vi "FindAllMessages.vi"(8 "error in (no error)":errorcluster, 11 "CS++Actor in":refnum<class "CS++Actor.lvclass">) -> (0 "error out":errorcluster, 3 "CS++Actor out":refnum<class "CS++Actor.lvclass">)   [LabVIEW 2014, in "CS++Actor.lvlib" / "CS++Actor.lvclass"]
doc: "Searches for all messages in this actor."
uses:
  CS++Actor.lvclass
  CS++Actor.lvclass/CS++Actor.ctl
  CSPP_Message/CS++Message.lvclass
  CSPP_Message/CS++Message.lvclass/CS++Message.ctl
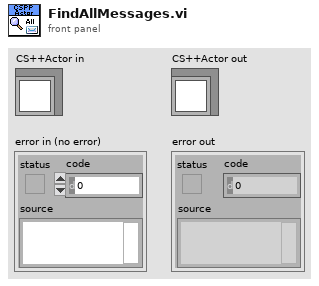
[diagram p1: front panel]
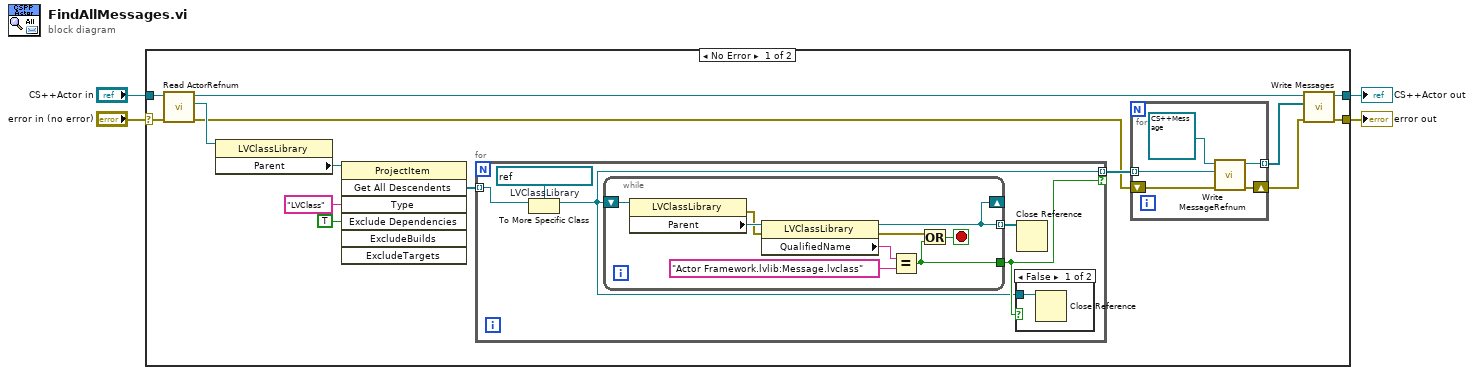
[diagram p0: block diagram]
diagram:
  n1 = case shown="No Error" "error in (no error)" {
    selector: "error in (no error)" -> [w13 w40]
    tunnel: [w8 w40] -> w3
    tunnel: [w6 w39] -> w1
    tunnel: "CS++Actor in" -> [w14 w39]
    frame No Error {
      n2 = call "Read ActorRefnum.vi"("error in (no error)"=w13, "CS++Actor in"=w14) -> ("error out"=w9:errorcluster, "ActorRefnum"=w12:refnum<vi>, "CS++Actor out"=w7:refnum<class "CS++Actor.lvclass">)  [unwired: 7 in]
      n3 = property class="LVClassLibrary"(reference=w12) -> ("Parent"=w16:refnum<vi>)  [unwired: 1 in, 2 out]
      n4 = invoke class="ProjectItem" method="Get All Descendents"(reference=w16, "Type"="LVClass", "Exclude Dependencies"=TRUE ("ExcludeDependencies")) -> ("All Descendents"=w15:refnum<vi>[])  [unwired: 4 in, 6 out]
      n5 = for {
        tunnel: w15 -> [w27] mode=indexing
        tunnel: [w24] -> w11 mode=indexing if=w25
        w28 = refnum<vi> refnum  # LVClassLibrary
        n6 = To More Specific Class(target class=w28, reference=w27) -> (specific class reference=w24:refnum<vi>)  [unwired: 1 in, 1 out]
        n7 = while {
          shift-right: [w32] -> _
          shift-left: w24 -> [w38]
          tunnel: [w32] -> w26 mode=indexing
          tunnel: [w31] -> w25
          stop <- w33 stop-if-true
          n8 = property class="LVClassLibrary"(reference=w38) -> (error out=w30:errorcluster, "Parent"=w34:refnum<vi>)  [unwired: 1 in, 1 out]
          n9 = property class="LVClassLibrary"(reference=w34, error in=w30) -> (reference out=w32:refnum<vi>, error out=w35:errorcluster, "QualifiedName"=w37:string)
          n10 = Equal?(x=w37, y="Actor Framework.lvlib:Message.lvclass") -> (x = y?=w31:bool)
          n11 = Or(x=w35, y=w31) -> (x .or. y?=w33:bool)
        }
        n12 = case shown="False" w25 {
          tunnel: w24 -> [w29 _]
          frame False {
            n13 = Close Reference(reference=w29) -> ()  [unwired: 1 in, 1 out]
          }
          frame True {
          }
        }
        n14 = Close Reference(reference=w26) -> ()  [unwired: 1 in, 1 out]
      }
      n15 = for {
        shift-right: [w23] -> w10
        shift-left: w9 -> [w22]
        tunnel: w11 -> [w21] mode=indexing
        tunnel: [w19] -> w5 mode=indexing
        n16 = call "Write MessageRefnum.vi"("error in (no error)"=w22, "MessageRefnum"=w21, "CS++Message in"=refnum<class "CS++Message.lvclass"> refnum ("CS++Message.lvlib:CS++Message.lvclass")) -> ("error out"=w23:errorcluster, "CS++Message out"=w19:refnum<class "CS++Message.lvclass">)  [unwired: 7 in]
      }
      n17 = call "Write Messages.vi"("error in (no error)"=w10, "Messages"=w5, "CS++Actor in"=w7) -> ("error out"=w8:errorcluster, "CS++Actor out"=w6:refnum<class "CS++Actor.lvclass">)  [unwired: 7 in]
    }
    frame Error {
    }
  }
  "error out" <- w3
  "CS++Actor out" <- w1
